vi "BRig_Host__Loop_Consumer_RunState__closedLoop_main.vi"(0 "input_idx":i32[](array[numeric]), 2 "input_module":string=" module1 ", 3 "input_forceUpdate":bool, 4 "input_updateTrial_first":u16, 5 "input_updateTrial_subsequent":u16, 6 "input_dataTS":u16[][](array[numeric]), 7 "input_updateID":u16, 8 "input_dataPlot":u16[][](array[numeric]), 9 "input_trialList":u16[](array[numeric]), 10 "input_dataLC":u16[](array[numeric]), 12 "input_dataExp":u16[](array[numeric])) -> (11 "output_trialList":u16[](array[numeric]), 13 "output_updateID":u16, 15 "output_cmdList":bool, 16 "output_cmdList":u16[][](array[numeric]), 17 "output_thres":bool, 18 "output_thres1":u16, 19 "output_thres2":u16)   [LabVIEW 2014]
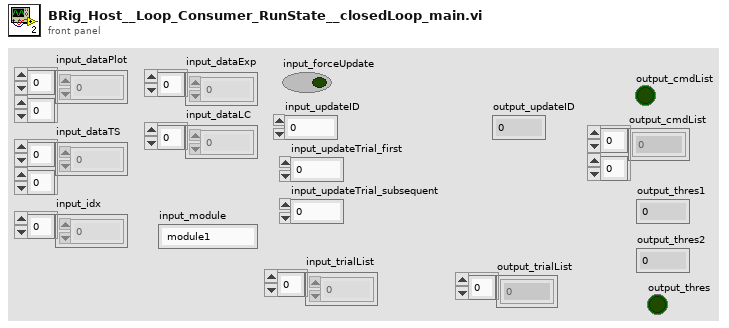
[diagram p1: front panel]
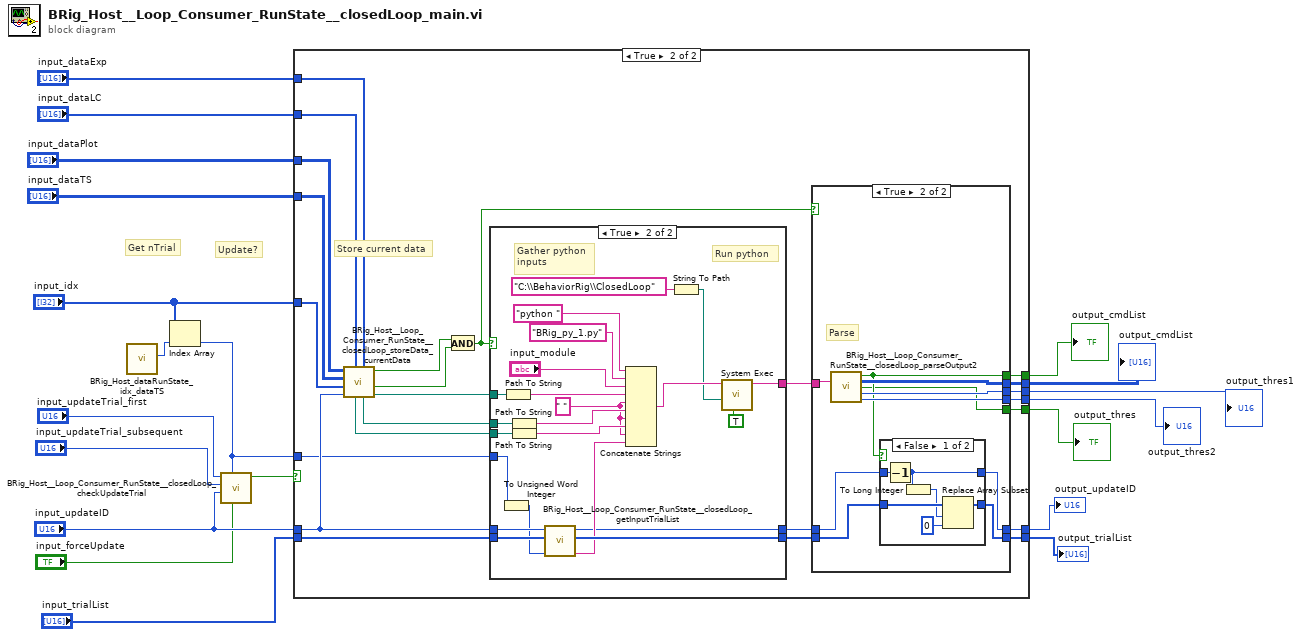
[diagram p0: block diagram]
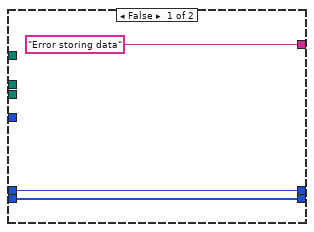
[diagram p5: hidden frame]
diagram:
  # "Update?"
  # "Get nTrial"
  n1 = call "BRig_Host_dataRunState_idx_dataTS.vi"() -> ("output_idx_dataTS"=w20:i32)  [unwired: 11 in]
  n2 = Index Array(array="input_idx", index=w20) -> (element=w14:i32)
  n3 = call "BRig_Host__Loop_Consumer_RunState__closedLoop_checkUpdateTrial.vi"("input_forceUpdate"="input_forceUpdate", "input_nTrial"=w14, "input_updateID"="input_updateID", "input_updateTrial_subsequent"="input_updateTrial_subsequent", "input_updateTrial_first"="input_updateTrial_first") -> ("output_update"=w13:bool)  [unwired: 6 in]
  n4 = case shown="True" w13 {
    tunnel: "input_idx" -> [_ w44]
    tunnel: w14 -> [_ w32]
    tunnel: "input_updateID" -> [w22 w36]
    tunnel: "input_dataPlot" -> [_ w46]
    tunnel: "input_dataTS" -> [_ w45]
    tunnel: [w22 w30] -> w10
    tunnel: "input_dataExp" -> [_ w39]
    tunnel: "input_dataLC" -> [_ w40]
    tunnel: "input_trialList" -> [w21 w33]
    tunnel: [w21 w28] -> w6
    tunnel: [_ w27] -> w5
    tunnel: [_ w26] -> w4
    tunnel: [_ w25] -> w3
    tunnel: [_ w24] -> w2
    tunnel: [_ w23] -> w1
    frame False {
    }
    frame True {
      # "Store current data"
      n5 = call "BRig_Host__Loop_Consumer_RunState__closedLoop_storeData_currentData.vi"("input_dataExp"=w39, "input_dataLC"=w40, "input_updateID"=w36, "input_idx"=w44, "input_dataTS"=w45, "input_dataPlot"=w46) -> ("output_filepath_dataTS"=w41:path, "output_dataTS"=w42:bool, "output_dataPlot"=w43:bool, "output_filepath_dataExp"=w38:path, "output_filepath_dataLC"=w37:path)  [unwired: 1 out]
      n6 = And(x=w43, y=w42) -> (x .and. y?=w35:bool)
      n7 = case shown="True" w35 {
        tunnel: w41 -> [_ w91]
        tunnel: w38 -> [_ w82]
        tunnel: w37 -> [_ w81]
        tunnel: w36 -> [w69 w76]
        tunnel: [w69 w70] -> w31
        tunnel: ["Error storing data" ("command line") w78] -> w34
        tunnel: w33 -> [w67 w75]
        tunnel: w32 -> [_ w74]
        tunnel: [w67 w72] -> w29
        frame False {
        }
        frame True {
          w77 = " "
          # "Run python"
          # "Gather python\ninputs"
          n8 = To Unsigned Word Integer(number=w74) -> (unsigned 16bit integer=w73:u16)
          n9 = Path To String(path=w91) -> (string=w90:string)
          n10 = Path To String(path=w82) -> (string=w80:string)
          n11 = Path To String(path=w81) -> (string=w79:string)
          n12 = call "BRig_Host__Loop_Consumer_RunState__closedLoop_getInputTrialList.vi"("input_nTrial"=w73, "input_trialList"=w75, "input_updateID"=w76) -> (0:"output_trialList"=w71:string, 2:"output_trialList"=w72:u16[], "output_updateID"=w70:u16)  [unwired: 6 in]
          n13 = Concatenate Strings("python " ("command line"), "BRig_py_1.py" ("command line"), "input_module", w90, w77, w80, w77, w79, w77, w71) -> (w85:string)
          n14 = String To Path(string="C:\\BehaviorRig\\ClosedLoop" ("command line")) -> (path=w83:path)
          n15 = call <vilib>:"System Exec.vi"("run minimized? (F)"=TRUE, "working directory"=w83, "command line"=w85) -> ("standard output"=w78:string)  [unwired: 5 in, 3 out]
        }
      }
      n16 = case shown="True" w35 {
        tunnel: w34 -> [_ w54]
        tunnel: w31 -> [w48 w58]
        tunnel: [w48 w55] -> w30
        tunnel: w29 -> [w47 w57]
        tunnel: [w47 w56] -> w28
        tunnel: [_ w50] -> w27
        tunnel: [_ w51] -> w26
        tunnel: [_ w52] -> w25
        tunnel: [_ w53] -> w24
        tunnel: [_ w49] -> w23
        frame False {
        }
        frame True {
          # "Parse"
          n17 = call "BRig_Host__Loop_Consumer_RunState__closedLoop_parseOutput2.vi"("String"=w54) -> ("output_cmd"=w50:bool, "output_cmdList"=w51:u16[][], "output_thres"=w49:bool, "output_thres1"=w52:u16, "output_thres2"=w53:u16)  [unwired: 10 in]
          n18 = case shown="False" w50 {
            tunnel: w58 -> [w64 w66]
            tunnel: w57 -> [w63 w65]
            tunnel: [w61 w66] -> w55
            tunnel: [w59 w65] -> w56
            frame False {
              n19 = Decrement(x=w64) -> (x-1=w61:u16)
              n20 = To Long Integer(number=w61) -> (32bit integer=w62:i32)
              n21 = Replace Array Subset(array=w63, new element=u16 0 ("new element/subarray"), index=w62) -> (w59:u16[])
            }
            frame True {
            }
          }
        }
      }
    }
  }
  "output_updateID" <- w10
  "output_trialList" <- w6
  "output_cmdList" <- w5
  "output_cmdList" <- w4
  "output_thres1" <- w3
  "output_thres2" <- w2
  "output_thres" <- w1
